vi "5. Sort Array.vi"() -> ()   [LabVIEW 2012]
panel:
  out "Square":dbl
  in  "Number":dbl
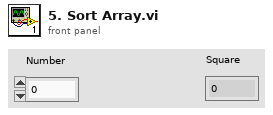
[diagram p1: front panel]
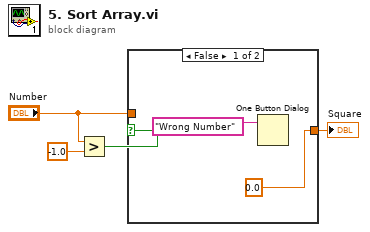
[diagram p0: block diagram]
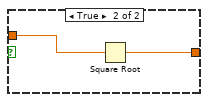
[diagram p2: hidden frame]
diagram:
  n1 = Greater?(x="Number", y=-1.0) -> (0:w3:bool)
  n2 = case shown="False" w3 {
    tunnel: "Number" -> [_ w8]
    tunnel: [0.0 w7] -> w1
    frame False {
      n3 = One Button Dialog(message="Wrong Number") -> ()  [unwired: 1 in, 1 out]
    }
    frame True {
      n4 = Square Root(x=w8) -> (sqrt(x)=w7:dbl)
    }
  }
  "Square" <- w1
